vi "MES操作函数 backup.vi"(3 "Tips":bool, 5 "测试结果":string="产品名称：SA 左前玻璃升降器\n测试程序版本：150113-A0\n测试时间：\n,,!测试步骤,判定条件,测试值!上电,-,电压：14.0V 限流：1.0A!软件版本号,{06 50 01 00 32 01 F4 AA;\n03 7F 2F 31 AA AA AA AA},06 50 01 00 32 01 F4 AA \n03 7F 2F 31 AA AA AA AA ;!中控锁上锁,{01 AA 02 A4 86 01 01},00 AA 02 A4 86 01 01 90 ，不合格!", 7 "SN":string="0105442MF011400002", 8 "error in (no error)":errorcluster caption="错误输入（无错误）", 10 "总结果（测试）":bool, 11 "MES配置":T2={"接口地址："="http://10.9.30.175:50100/manufacturing/IntegrationServlet?InterType=XML&message=", "SITE（站点）   "="A157", "PWD（口令）"="123456", "RESOURCE（资源）"="A-6-Z-TEST", "OPERATION（工序）"="Z-TEST", "USER（用户）"="TEST", "QTY"="", "ACTIVITY"="", "NC_CODE（NG代码）"="", "启用MES"=TRUE}) -> (0 "error out":errorcluster caption="错误输出", 2 "Data(OUT)":string="http://10.9.30.175:50100/manufacturing/IntegrationServlet?InterType=XML&message= ERROR<PRODUCTION_REQUEST><NC_LOG_COMPLETE><SITE>A157</SITE><OWNER TYPE=\"USER\">TEST</OWNER><NC_CONTEXT>0105442MF011400002</NC_CONTEXT><QTY></QTY><IDENTIFIER></IDENTIFIER><FAILURE_ID></FAILURE_ID><DEFECT_COUNT>1</DEFECT_COUNT><COMMENTS></COMMENTS><DATE_TIME></DATE_TIME><RESOURCE>A-6-Z-TEST</RESOURCE><OPERATION>Z-TEST</OPERATION><ROOT_CAUSE_OPER></ROOT_CAUSE_OPER><NC_CODE></NC_CODE><ACTIVITY></ACTIVITY></NC_LOG_COMPLETE></PRODUCTION_REQUEST>!erpautogy03!1234567@byd!ERROR,测试文件11V1.0,测试程序11V1.0!产品名称：SA 左前玻璃升降器\n测试程序版本：150113-A0\n测试时间：\n,,!测试步骤,判定条件,测试值!上电,-,电压：14.0V 限流：1.0A!软件版本号,{06 50 01 00 32 01 F4 AA;\n03 7F 2F 31 AA AA AA AA},06 50 01 00 32 01 F4 AA \n03 7F 2F 31 AA AA AA AA ;!中控锁上锁,{01 AA 02 A4 86 01 01},00 AA 02 A4 86 01 01 90 ，不合格!")   [LabVIEW 2011]
panel:
  out "输出簇":T1
  out "数组":string[](array[string])
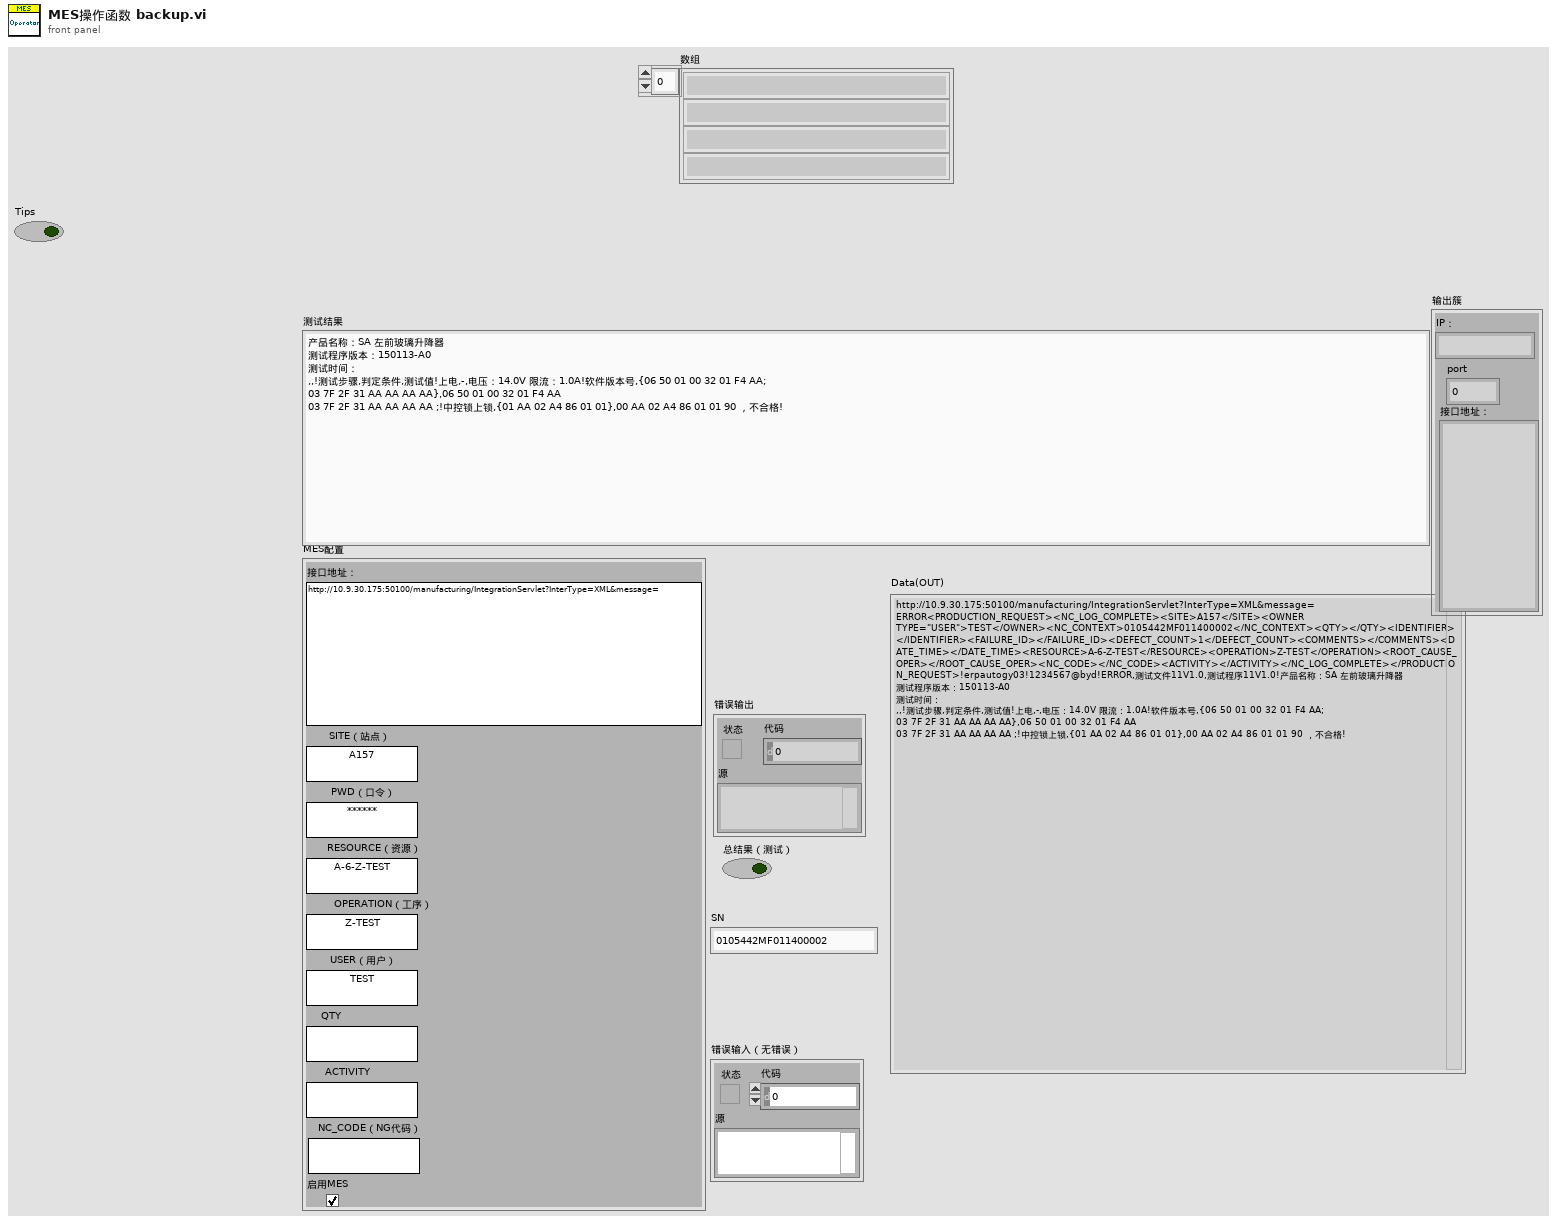
[diagram p1: front panel]
types:
  T1 = cluster{"IP：":string, "port":i32, "接口地址：":string}
  T2 = typedef "MES设置.ctl" = cluster{"接口地址：":string, "SITE（站点）   ":string, "PWD（口令）":string, "RESOURCE（资源）":string, "OPERATION（工序）":string, "USER（用户）":string, "QTY":string, "ACTIVITY":string, "NC_CODE（NG代码）":string, "启用MES":bool}
  T3 = enum16{"USER_CHECK", "SFC_CHECK", "RLT_PASS", "RLT_ERROR", "RES_AREA"}
  T4 = enum16{"open", "replace", "create", "open or create", "replace or create", "replace or create with confirmation"}
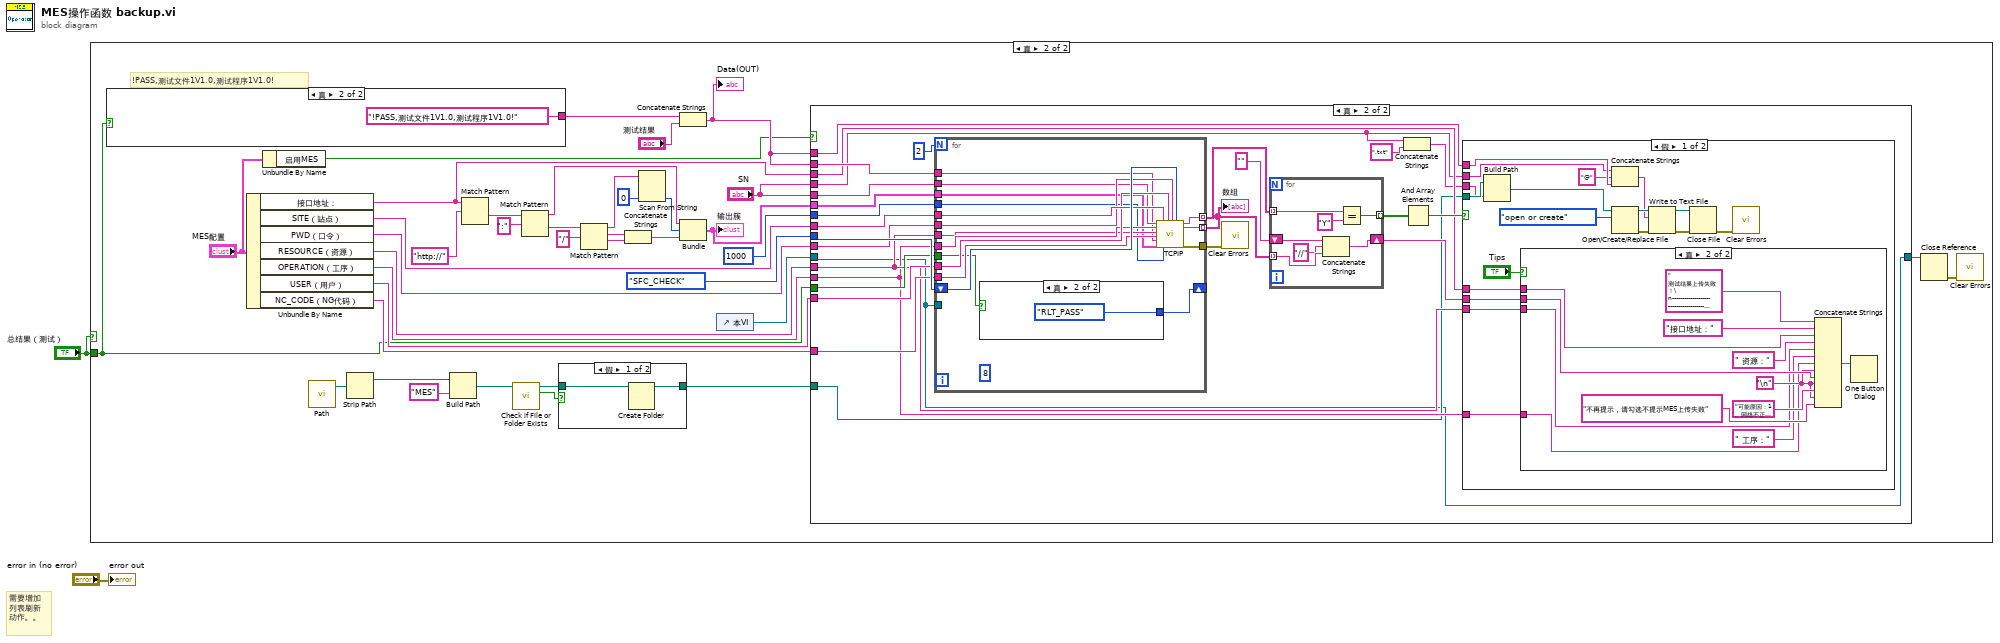
[diagram p0: block diagram]
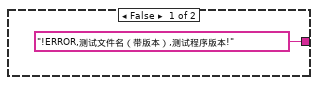
[diagram p4: hidden frame]
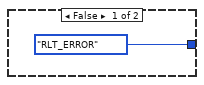
[diagram p8: hidden frame]
diagram:
  # "需要增加\n列表刷新\n动作。。"
  n1 = case shown="真" "总结果（测试）" {
    tunnel: "总结果（测试）" -> [_ w22]
    frame False {
    }
    frame True {
      # "!PASS,测试文件1V1.0,测试程序1V1.0!"
      n2 = case shown="真" w22 {
        tunnel: ["!ERROR,测试文件名（带版本）,测试程序版本!" ("字符串") "!PASS,测试文件1V1.0,测试程序1V1.0!" ("字符串")] -> w21
        frame False {
        }
        frame True {
        }
      }
      n3 = Unbundle By Name("MES配置") -> ("接口地址："=w18:string, "SITE（站点）"=w39:string, "PWD（口令）"=w37:string, "RESOURCE（资源）"=w17:string, "OPERATION（工序）"=w36:string, "USER（用户）"=w38:string, "NC_CODE（NG代码）"=w35:string)
      n4 = Unbundle By Name("MES配置") -> ("启用MES"=w6:bool)
      n5 = call "Path.vi"() -> ("appended path"=w11:path)  [unwired: 11 in]
      n6 = Strip Path(path=w11) -> (stripped path=w12:path)  [unwired: 1 out]
      n7 = Build Path(base path=w12, name or relative path="MES" ("名称或相对路径")) -> (appended path=w14:path)
      n8 = Match Pattern(string=w18, regular expression="http://" ("正则表达式")) -> (after substring=w31:string)  [unwired: 1 in, 3 out]
      n9 = call <vilib>:"Check if File or Folder Exists.vi"("path"=w14) -> ("file or folder exists?"=w15:bool, "dup path"=w16:path)  [unwired: 8 in, 1 out]
      n10 = Match Pattern(string=w31, regular expression=":" ("正则表达式")) -> (before substring=w26:string, after substring=w29:string)  [unwired: 1 in, 2 out]
      n11 = case shown="假" w15 {
        tunnel: w16 -> [w42 w44]
        tunnel: [w43 w44] -> w10
        frame False {
          n12 = Create Folder(path (use dialog)=w42) -> (created path=w43:path)  [unwired: 2 in, 2 out]
        }
        frame True {
        }
      }
      n13 = Match Pattern(string=w29, regular expression="/" ("正则表达式")) -> (before substring=w27:string, match substring=w3:string, after substring=w5:string)  [unwired: 1 in, 1 out]
      n14 = Concatenate Strings(w3, w5) -> (w4:string)
      n15 = Scan From String(input string=w27, default 1=0 ("默认值 1")) -> (output 1=w24:i32)  [unwired: 3 in, 3 out]
      n16 = Concatenate Strings(w21, "测试结果") -> (w20:string)
      "Data(OUT)" <- w20
      n17 = Bundle("接口地址："=w26, "默认值 1"=w24, w4) -> (w25:cluster{"接口地址：":string, "默认值 1":i32, string})  [unwired: 1 in]
      "输出簇" <- w25
      n18 = control-ref of="本VI"() -> (w9:refnum<vi>)
      n19 = case shown="真" w6 {
        tunnel: T3."SFC_CHECK" ("STATE") -> [_ w74]
        tunnel: w39 -> [_ w73]
        tunnel: w38 -> [_ w72]
        tunnel: w37 -> [_ w71]
        tunnel: "SN" -> [_ w70]
        tunnel: w36 -> [_ w52]
        tunnel: w35 -> [_ w69]
        tunnel: u64 1000 ("TCP超时") -> [_ w68]
        tunnel: w20 -> [_ w67]
        tunnel: w25 -> [_ w66]
        tunnel: w22 -> [_ w64]
        tunnel: w20 -> [_ w57]
        tunnel: "SN" -> [_ w49]
        tunnel: w18 -> [_ w54]
        tunnel: w17 -> [_ w53]
        tunnel: w9 -> [w47 w50]
        tunnel: w10 -> [_ w51]
        tunnel: [w47 w50] -> w8
        frame False {
        }
        frame True {
          n20 = for {
            N: 2 -> [_]
            tunnel: w73 -> [w126]
            tunnel: w72 -> [w125]
            tunnel: w71 -> [w124]
            tunnel: w70 -> [w123]
            tunnel: w52 -> [w122]
            tunnel: w53 -> [w121]
            tunnel: w69 -> [w120]
            tunnel: w68 -> [w119]
            tunnel: w67 -> [w118]
            tunnel: w66 -> [w117]
            shift-right: [w115] -> _
            shift-left: w74 -> [w127]
            tunnel: w64 -> [w116]
            tunnel: [w114] -> w60 mode=indexing
            tunnel: [w113] -> w63 mode=indexing
            tunnel: [w112] -> w55
            tunnel: w50 -> [_]
            (unwired) 8 ("图像深度")
            n21 = case shown="真" w116 {
              tunnel: [T3."RLT_ERROR" ("STATE") T3."RLT_PASS" ("STATE")] -> w115
              frame False {
              }
              frame True {
              }
            }
            n22 = call "TCPIP.vi"("SFC"=w123, "OPERATOR"=w122, "RESOURCE"=w121, "NC_CODE"=w120, "TESTRLT"=w118, "SERVER"=w117, "SITE"=w126, "TCP超时"=w119, "USER"=w125, "PWD"=w124, "STATE"=w127) -> ("Y&N"=w113:string, "系统消息"=w114:string, "error out"=w112:errorcluster)  [unwired: 6 in]
          }
          "数组" <- w60
          n23 = call <vilib>:"Clear Errors.vi"("error in (no error)"=w55) -> ()  [unwired: 6 in, 1 out]
          n24 = for {
            tunnel: w63 -> [w111] mode=indexing
            tunnel: [w109] -> w62 mode=indexing
            tunnel: w60 -> [w108] mode=indexing
            shift-right: [w107] -> w58
            shift-left: "" -> [w106]
            n25 = Concatenate Strings(w106, "//" ("字符串"), w108) -> (w107:string)
            n26 = Equal?(x=w111, y="Y") -> (x = y?=w109:bool)
          }
          n27 = Concatenate Strings(w49, ".txt" ("字符串")) -> (w48:string)
          n28 = And Array Elements(Boolean array=w62) -> (logical AND=w61:bool)
          n29 = case shown="假" w61 {
            tunnel: w58 -> [w92 _]
            tunnel: w57 -> [w83 _]
            tunnel: w49 -> [w82 _]
            tunnel: w54 -> [w79 _]
            tunnel: w53 -> [w78 _]
            tunnel: w52 -> [w77 _]
            tunnel: w51 -> [w76 _]
            tunnel: w48 -> [w75 _]
            frame False {
              n30 = Build Path(base path=w76, name or relative path=w75) -> (appended path=w90:path)
              n31 = case shown="真" "Tips" {
                tunnel: w92 -> [_ w103]
                tunnel: w79 -> [_ w97]
                tunnel: w78 -> [_ w95]
                tunnel: w77 -> [_ w93]
                frame False {
                }
                frame True {
                  w101 = "\n"
                  n32 = Concatenate Strings("                  测试结果上传失败！\n---------------------------------------------\n", "接口地址：" ("字符串"), w97, " 资源：" ("字符串"), w95, " 工序：" ("字符串"), w93, w101, w103, w101, "可能原因：1、网络不正确；2、配置参数错误；3、条码错误；4、SFC未维护。" ("字符串"), w101, "不再提示，请勾选不提示MES上传失败" ("字符串")) -> (w104:string)
                  n33 = One Button Dialog(message=w104) -> ()  [unwired: 1 in, 1 out]
                }
              }
              n34 = Concatenate Strings(w82, "@" ("字符串"), w83) -> (w80:string)
              n35 = Open/Create/Replace File(file path (use dialog)=w90, operation (0:open)=T4."open or create" ("操作(0:open)")) -> (refnum out=w88:refnum<file>, error out=w87:errorcluster)  [unwired: 4 in, 1 out]
              n36 = Write to Text File(file (use dialog)=w88, text=w80, error in=w87) -> (refnum out=w85:refnum<file>, error out=w86:errorcluster)  [unwired: 1 in, 1 out]
              n37 = Close File(refnum=w85, error in=w86) -> (error out=w84:errorcluster)  [unwired: 1 out]
              n38 = call <vilib>:"Clear Errors.vi"("error in (no error)"=w84) -> ()  [unwired: 6 in, 1 out]
            }
            frame True {
            }
          }
        }
      }
      n39 = Close Reference(reference=w8) -> (error out=w7:errorcluster)  [unwired: 1 in]
      n40 = call <vilib>:"Clear Errors.vi"("error in (no error)"=w7) -> ()  [unwired: 6 in, 1 out]
    }
  }
  "error out" <- "error in (no error)"
